vi "ArrayMinMaxCalibracao.vi"() -> (0 "max":dbl[](array[numeric]), 1 "min":dbl[](array[numeric]))   [LabVIEW 2019]
uses:
  <vilib>/Utility/file.llb/Read Delimited Spreadsheet (DBL).vi
panel:
  out "input":dbl[](array[numeric])
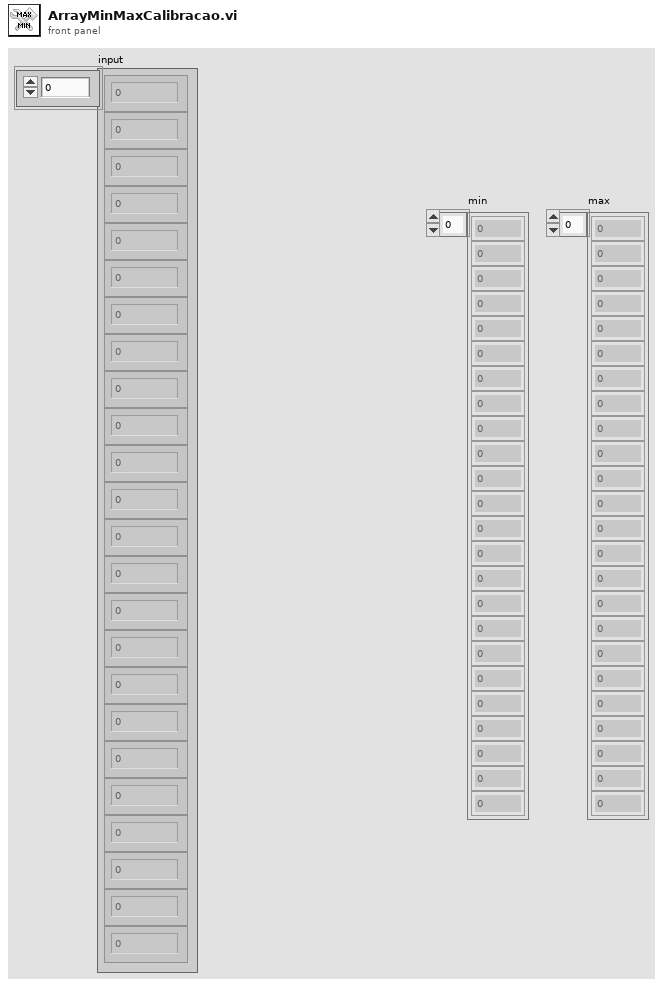
[diagram p1: front panel]
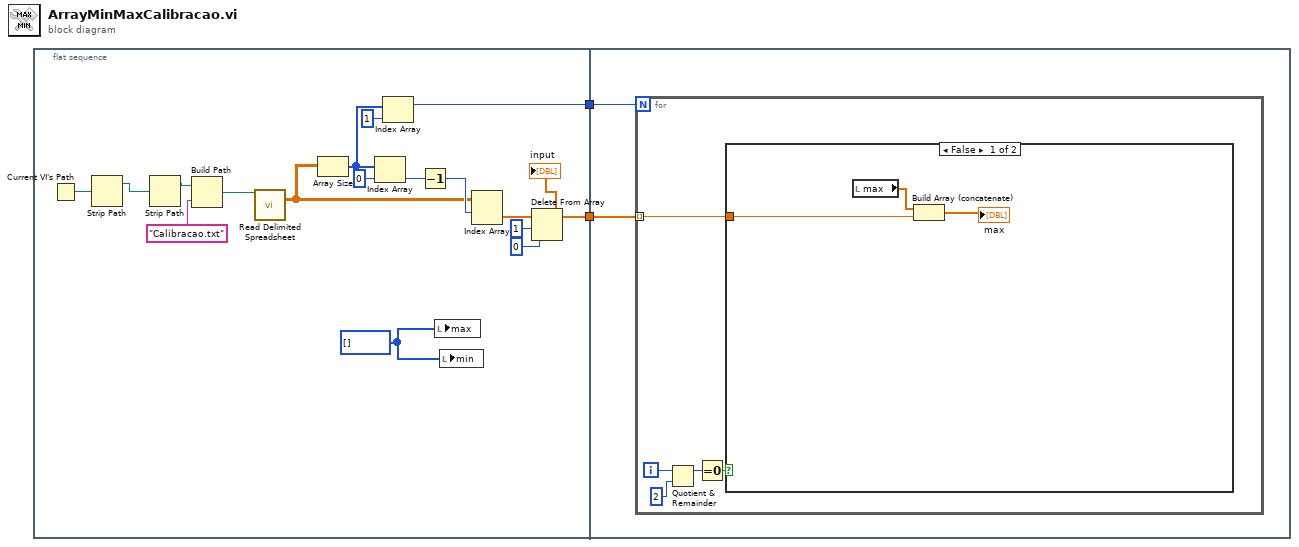
[diagram p0: block diagram]
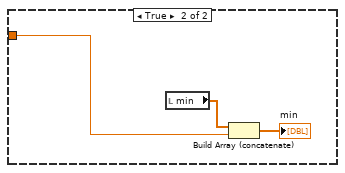
[diagram p2: hidden frame]
diagram:
  n1 = flat-sequence {
    tunnel: [w10] -> w2
    tunnel: [w6] -> w1
    tunnel: w2 -> [w21]
    tunnel: w1 -> [w20]
    frame #0 {
      w11 = i32[] [] ("max")
      n2 = Current VI's Path() -> (path=w14:path)
      n3 = Strip Path(path=w14) -> (stripped path=w15:path)  [unwired: 1 out]
      n4 = Strip Path(path=w15) -> (stripped path=w12:path)  [unwired: 1 out]
      n5 = Build Path(base path=w12, name or relative path="Calibracao.txt") -> (appended path=w13:path)
      n6 = call-poly <vilib>:"Read Delimited Spreadsheet.vi"("file path (dialog if empty)"=w13) -> ("all rows"=w16:dbl[][])  [unwired: 9 in, 5 out]
      n7 = Array Size(array=w16) -> (size(s)=w8:i32[])
      n8 = Index Array(array=w8, index=0) -> (element=w4:i32)
      n9 = Index Array(array=w8, index=1) -> (element=w10:i32)
      n10 = Decrement(x=w4) -> (x-1=w17:i32)
      n11 = local write "max"(w11) -> ()
      n12 = local write "min"(w11) -> ()
      n13 = Index Array(array=w16, index (row)=w17) -> (element=w7:dbl[])  [unwired: 1 in]
      n14 = Delete From Array(array=w7, length=1, index=0) -> (array with subset deleted=w6:dbl[])  [unwired: 1 out]
      "input" <- w6
    }
    frame #1 {
      n15 = for {
        N: w21 -> [_]
        tunnel: w20 -> [w22] mode=indexing
        i -> [w26]
        n16 = Quotient & Remainder(x=w26, y=2) -> (x-y*floor(x/y)=w24:i32)  [unwired: 1 out]
        n17 = Equal To 0?(x=w24) -> (x = 0?=w23:bool)
        n18 = case shown="False" w23 {
          tunnel: w22 -> [w27 w31]
          frame False {
            n19 = local read "max"() -> (w29:dbl[])
            n20 = Build Array (concatenate)(w29, w27) -> (→"max":dbl[])
          }
          frame True {
            n21 = local read "min"() -> (w30:dbl[])
            n22 = Build Array (concatenate)(w30, w31) -> (→"min":dbl[])
          }
        }
      }
    }
  }
